vi "Setup DecFrame Data.vi"(6 "Border Spacing":i16=-2, 7 "Monitor Select":T1, 8 "Error":errorcluster, 9 "FPLocation":T2=enum."MID-CTR", 10 "Decoration Index":i32, 11 "FP":refnum<class "DecFrame_FP.lvclass">) -> (0 "Error Out":errorcluster, 3 "FP Out":refnum<class "DecFrame_FP.lvclass">)   [LabVIEW 2024, in "DecFrame_FP.lvclass"]
uses:
  DecFrame_FP.lvclass
  TypeDefs_Utility/ENUM RB_Pos_Quadrant Position.ctl
  TypeDefs_Utility/ENUM_Monitor Select.ctl
  DecFrame_FP.lvclass/DecFrame_FP.ctl
  FP/FP.lvclass
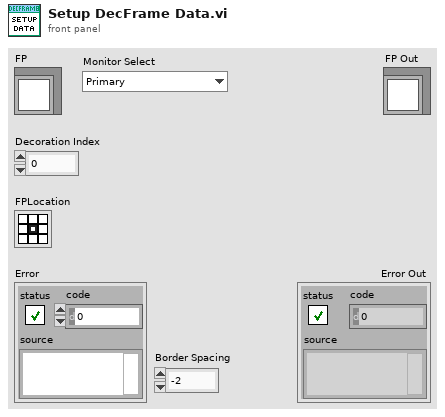
[diagram p1: front panel]
types:
  T1 = typedef "ENUM_Monitor Select.ctl" = enum16{"Primary", "Secondary (Right first)", "Right of Primary", "Left of Primary", "Above Primary", "Below Primary"}
  T2 = typedef "ENUM RB_Pos_Quadrant Position.ctl" = enum32{"LFT-TOP", "MID-TOP", "RGT-TOP", "LFT-CTR", "MID-CTR", "RGT-CTR", "LFT-BOT", "MID-BOT", "RGT-BOT"}
  T3 = cluster{"Left":i16, "Top":i16, "Right":i16, "Bottom":i16}
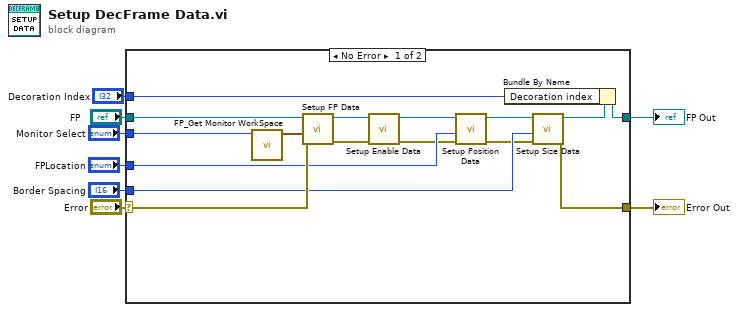
[diagram p0: block diagram]
diagram:
  n1 = case shown="No Error" "Error" {
    selector: "Error" -> [w23 w26]
    tunnel: [w11 w26] -> w7
    tunnel: [w17 w25] -> w5
    tunnel: "FP" -> [w24 w25]
    tunnel: "FPLocation" -> [w19 _]
    tunnel: "Decoration Index" -> [w16 _]
    tunnel: "Border Spacing" -> [w13 _]
    tunnel: "Monitor Select" -> [w9 _]
    frame No Error {
      n2 = call "FP_Get Monitor WorkSpace.vi"("Monitor Select"=w9) -> ("Selected Work Space Out"=w10:T3)  [unwired: 7 in, 3 out]
      n3 = call "Setup FP Data.vi"("Error"=w23, "WkSpace"=w10, "FP"=w24) -> ("Error Out"=w22:errorcluster, "FP Out"=w21:refnum<class "DecFrame_FP.lvclass">)  [unwired: 7 in]
      n4 = call-dynamic "Setup Enable Data.vi"("Error"=w22, "FP"=w21) -> ("Error Out"=w18:errorcluster, "FP Out"=w20:refnum<class "DecFrame_FP.lvclass">)  [unwired: 8 in]
      n5 = call-dynamic "Setup Position Data.vi"("Error"=w18, "FPLocation"=w19, "FP"=w20) -> ("Error Out"=w12:errorcluster, "FP Out"=w15:refnum<class "DecFrame_FP.lvclass">)  [unwired: 7 in]
      n6 = call-dynamic "Setup Size Data.vi"("Error"=w12, "Border Spacing"=w13, "FP"=w15) -> ("Error Out"=w11:errorcluster, "FP Out"=w14:refnum<class "DecFrame_FP.lvclass">)  [unwired: 7 in]
      n7 = Bundle By Name(cluster=w14, "Decoration index"=w16) -> (w17:refnum<class "DecFrame_FP.lvclass">)
    }
    frame Error {
    }
  }
  "Error Out" <- w7
  "FP Out" <- w5
